vi "Uninstall Dependencies.vi"(0 "NIPKG_LV in":refnum<class "NIPKG_LV.lvclass">) -> (4 "NIPKG_LV out":refnum<class "NIPKG_LV.lvclass">)   [LabVIEW 2017, in "CL_G3_VIComponentBuilder.lvlib" / "NIPKG_LV.lvclass"]
doc: "Uninstalls the dependencies specified by this export at build time."
uses:
  NIPKG_LV.lvclass
  C:/Tool Chain Support/Software Module Builder/Source/Exports/Exports/Export.lvclass
  Exports/Export.lvclass/Export.ctl
  NIPKG_LV.lvclass/NIPKG_LV.ctl
  Exports/Accessors/Write Export Operation Errors.vi
  Exports/Accessors/Read Export Operation Errors.vi
  Exports/Accessors/Read Built Export's Full Path.vi
  Accessors/Read Build Machine Feed Folderpath.vi
  <vilib>/National Instruments/NIPM API (Beta)/NIPM_API.lvlib
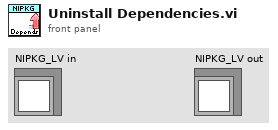
[diagram p1: front panel]
types:
  T1 = typedef "NIPM_API.lvlib/package attributes.ctl" = cluster{"Package Name":string, "Display name":string, "Version":string, "Display version":string, "Synopsis":string, "Description":string, "Maintainer":string, "Maintainer email address":string, "Category":string, "Homepage":string, "Release notes":string, "Depends":string[], "Recommends":string[], "Suggests":string[], "Conflicts":string[], "Provides":string[], "Replaces":string[], "Supplements":string[], "Enhances":string[], "Product":bool, "User visible":bool, "Installed size (KB)":u64, "Package filesize (bytes)":u64, "Architecture":string, "Agent":string, "MD5Checksum":string}
  T2 = typedef "NIPM_API.lvlib/feed.ctl" = cluster{"Name":string, "URI":string}
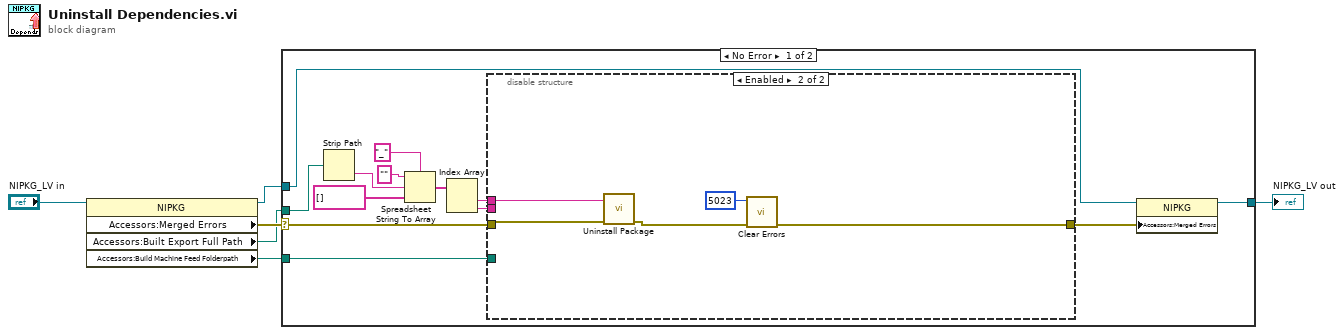
[diagram p0: block diagram]
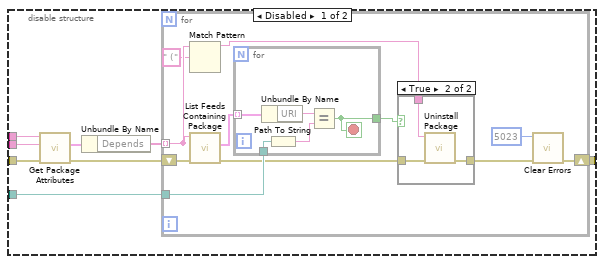
[diagram p2: hidden frame]
diagram:
  n1 = property class="NIPKG"(reference="NIPKG_LV in") -> (reference out=w3:refnum<class "NIPKG_LV.lvclass">, "Accessors:Merged Errors"=w5:errorcluster, "Accessors:Built Export Full Path"=w2:path, "Accessors:Build Machine Feed Folderpath"=w1:path)  [unwired: 1 in, 1 out]
  n2 = case shown="No Error" w5 {
    selector: w5 -> [w8 _]
    tunnel: [w18 w53] -> w4
    tunnel: w3 -> [w19 w53]
    tunnel: w2 -> [w17 _]
    tunnel: w1 -> [w9 _]
    frame No Error {
      n3 = Strip Path(path=w17) -> (name=w15:string)  [unwired: 1 out]
      n4 = Spreadsheet String To Array(delimiter (Tab)="_", format string="", spreadsheet string=w15, array type (2D Dbl)=string[] []) -> (array=w12:string[])
      n5 = Index Array(array=w12) -> (element #1=w11:string, element #2=w10:string)  [unwired: 2 in]
      n6 = disable-structure shown="Enabled" {
        disable-tunnel: w11 -> [w27 w52]
        disable-tunnel: w10 -> [w24 _]
        disable-tunnel: w9 -> [w23 _]
        disable-tunnel: w8 -> [w22 w51]
        disable-tunnel: [w20 w48] -> w7
        frame Disabled {
          n7 = call <vilib>:"Get Package Attributes.vi"("error in"=w22, "version"=w24, "package name"=w27) -> ("error out"=w21:errorcluster, "package attributes"=w26:T1)  [unwired: 5 in, 2 out]
          n8 = Unbundle By Name(w26) -> ("Depends"=w25:string[])
          n9 = for {
            tunnel: w25 -> [w30] mode=indexing
            tunnel: w23 -> [w37]
            shift-right: [w31] -> w20
            shift-left: w21 -> [w35]
            n10 = Match Pattern(string=w30, regular expression=" (") -> (before substring=w28:string)  [unwired: 1 in, 3 out]
            n11 = call <vilib>:"List Feeds Containing Package.vi"("error in"=w35, "package name"=w30) -> ("error out"=w34:errorcluster, "feeds"=w38:T2[])  [unwired: 8 in]
            n12 = for {
              tunnel: w38 -> [w47] mode=indexing
              tunnel: w37 -> [w46]
              tunnel: [w45] -> w36
              stop <- w45 stop-if-true
              n13 = Unbundle By Name(w47) -> ("URI"=w44:string)
              n14 = Path To String(path=w46) -> (string=w43:string)
              n15 = Equal?(x=w44, y=w43) -> (x = y?=w45:bool)
            }
            n16 = case shown="True" w36 {
              tunnel: w34 -> [w39 w42]
              tunnel: [w39 w41] -> w32
              tunnel: w28 -> [_ w40]
              frame False {
              }
              frame True {
                n17 = call <vilib>:"Uninstall Package.vi"("error in"=w42, "package name"=w40) -> ("error out"=w41:errorcluster)  [unwired: 8 in, 1 out]
              }
            }
            n18 = call <vilib>:"Clear Errors.vi"("error in (no error)"=w32, "specific error code to clear (0: all)"=5023) -> ("error out"=w31:errorcluster)  [unwired: 4 in, 1 out]
          }
        }
        frame Enabled {
          n19 = call <vilib>:"Uninstall Package.vi"("error in"=w51, "package name"=w52) -> ("error out"=w49:errorcluster)  [unwired: 8 in, 1 out]
          n20 = call <vilib>:"Clear Errors.vi"("error in (no error)"=w49, "specific error code to clear (0: all)"=5023) -> ("error out"=w48:errorcluster)  [unwired: 4 in, 1 out]
        }
      }
      n21 = property class="NIPKG"(reference=w19, "Accessors:Merged Errors"=w7) -> (reference out=w18:refnum<class "NIPKG_LV.lvclass">)  [unwired: 1 in, 1 out]
    }
    frame Error {
    }
  }
  "NIPKG_LV out" <- w4
